vi "MatchesToGlobalRect.vi"(11 "Matches":T2(array[cluster]) {"Bounding Box"."y" format="%.2f"; "Bounding Box"."x" format="%.2f"; "Position"."y" format="%.2f"; "Position"."x" format="%.2f"; "Score" format="%.2f"; "Scale" format="%.2f"; "Angle" format="%.2f"}) -> (3 "Global Rectangle":T1)   [LabVIEW 2013]
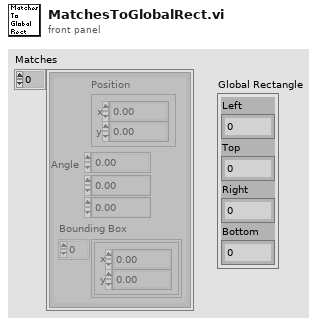
[diagram p1: front panel]
types:
  T1 = cluster{"Left":sgl, "Top":sgl, "Right":sgl, "Bottom":sgl}
  T2 = cluster{"Position":cluster{"x":sgl, "y":sgl}, "Angle":sgl, "Scale":sgl, "Score":sgl, "Bounding Box":cluster{"x":sgl, "y":sgl}[]}[]
  T3 = cluster{"Position":cluster{"x":sgl, "y":sgl}, "Angle":sgl, "Scale":sgl, "Score":sgl, "Bounding Box":cluster{"x":sgl, "y":sgl}[]}
  T4 = cluster{"Bounding Box[0]":cluster{"x":sgl, "y":sgl}, "Bounding Box[1]":cluster{"x":sgl, "y":sgl}, "Bounding Box[2]":cluster{"x":sgl, "y":sgl}, "Bounding Box[3]":cluster{"x":sgl, "y":sgl}, "Bounding Box[4]":cluster{"x":sgl, "y":sgl}, "Bounding Box[5]":cluster{"x":sgl, "y":sgl}, "Bounding Box[6]":cluster{"x":sgl, "y":sgl}, "Bounding Box[7]":cluster{"x":sgl, "y":sgl}, "Bounding Box[8]":cluster{"x":sgl, "y":sgl}}
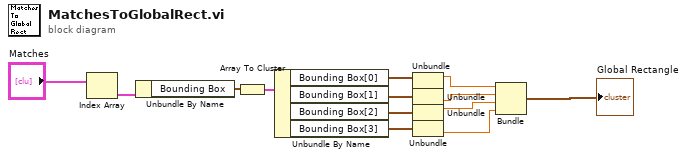
[diagram p0: block diagram]
diagram:
  n1 = Index Array(array="Matches") -> (element=w11:T3)  [unwired: 1 in]
  n2 = Unbundle By Name(w11) -> ("Bounding Box"=w10:cluster{"x":sgl, "y":sgl}[])
  n3 = Array To Cluster(array=w10) -> (cluster=w13:T4)
  n4 = Unbundle By Name(w13) -> ("Bounding Box[0]"=w9:cluster{"x":sgl, "y":sgl}, "Bounding Box[1]"=w8:cluster{"x":sgl, "y":sgl}, "Bounding Box[2]"=w5:cluster{"x":sgl, "y":sgl}, "Bounding Box[3]"=w4:cluster{"x":sgl, "y":sgl})
  n5 = Unbundle(w9) -> ("x"=w7:sgl)  [unwired: 1 out]
  n6 = Unbundle(w8) -> ("y"=w6:sgl)  [unwired: 1 out]
  n7 = Unbundle(w5) -> ("x"=w3:sgl)  [unwired: 1 out]
  n8 = Unbundle(w4) -> ("y"=w2:sgl)  [unwired: 1 out]
  n9 = Bundle("x"=w7, "y"=w6, "x"=w3, "y"=w2) -> (→"Global Rectangle":cluster{"x":sgl, "y":sgl, "x":sgl, "y":sgl})  [unwired: 1 in]
